vi "Template_Variables.vi"() -> (0 "Variable Names":string[](array[string]))   [LabVIEW 2010]
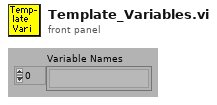
[diagram p1: front panel]
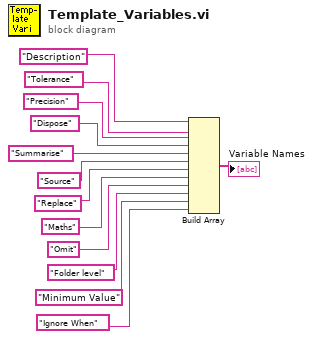
[diagram p0: block diagram]
diagram:
  n1 = Build Array("Description", "Tolerance", "Precision", "Dispose", "Summarise", "Source", "Replace", "Maths", "Omit", "Folder level", "Minimum Value", "Ignore When") -> (→"Variable Names":string[])
